vi "DispMsg.vi"(8 "错误输入（无错误）":errorcluster, 11 "nMsgType":i32) -> (0 "错误输出":errorcluster, 3 "返回类型":i32)   [LabVIEW 2014]
uses:
  X86Dll/ZXUTConfigMgr.dll
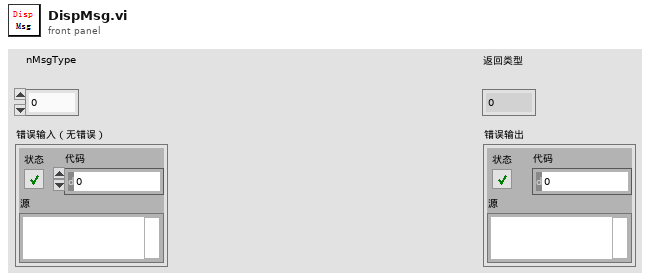
[diagram p1: front panel]
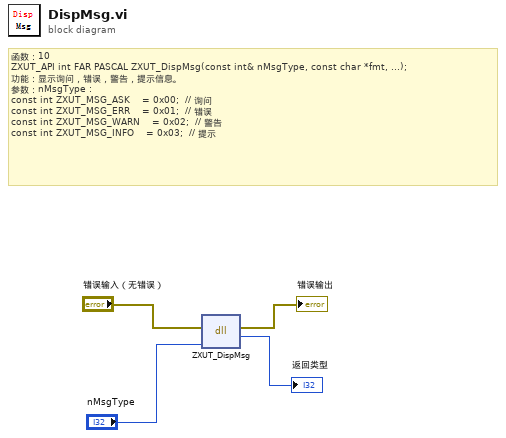
[diagram p0: block diagram]
diagram:
  # "函数：10\nZXUT_API int\tFAR PASCAL ZXUT_DispMsg(const int& nMsgType, const char *fmt, ...);\n功能：显示询问，错误，警告，提示信息。\n参数：nMsgType :\nconst int ZXUT_MSG_ASK\t\t\t\t= 0x00;\t\t// 询问\nconst int ZXUT_MSG_ERR\t\t\t\t= 0x01;\t\t// 错误\nconst int ZXUT_MSG_WARN\t\t\t\t= 0x02;\t\t// 警告\nconst int ZXUT_MSG_INFO\t\t\t\t= 0x03;\t\t// 提示"
  n1 = dll-call lib="D:/Software/Utrasonic on-line monitoring/X86Dll/ZXUTConfigMgr.dll" fn="ZXUT_DispMsg"(error in="错误输入（无错误）", "nMsgType"="nMsgType") -> (error out=→"错误输出":errorcluster, "返回类型"=→"返回类型":i32)  [unwired: 3 in, 1 out]
